vi "SVFA Frequency Response Subset (Real-Im).vi"(0 "stimulus signal X [EUx]":waveform(dbl)={"t0"=timestamp(0 s since 1904-01-01), "dt"=1e-05, "Y"=[]}, 1 "response signal Y [EUy]":waveform(dbl)={"t0"=timestamp(0 s since 1904-01-01), "dt"=1e-05, "Y"=[]}, 2 "window":T9=1 items=["None"=0, "Hanning"=1, "Hamming"=2, "Blackman-Harris"=3, "Exact Blackman"=4, "Blackman"=5, "Flat Top"=6, "4 Term B-Harris "=7, "7 Term B-Harris"=8, "Low Sidelobe"=9, "Force - Exponential"=10, "Blackman Nuttall"=11, "Triangle"=30, "Bartlett-Hanning"=31, "Bohman"=32, "Parzen"=33, "Welch"=34, "Kaiser"=60, "Dolph-Chebyshev"=61, "Gaussian"=62], 3 "frequency range":T7={"start frequency"=1000.0, "stop frequency"=5000.0} {"stop frequency" min=0.0 format="%.2f"; "start frequency" min=0.0 format="%.2f"}, 5 "error in (no error)":errorcluster, 6 "FRF mode":enum16{"H1", "H2", "H3"}(ring), 7 "averaging parameters":T10={"averaging mode"=enum."No averaging", "weighting mode"=enum."Exponential", "number of averages"=10, "linear mode"=enum."One shot"}, 8 "force/exp settings":T8={"force window [%]"=50.0, "exp window [%]"=10.0} {"exp window [%]" min=0.0 max=100.0 format="%.2f"; "force window [%]" min=0.0 max=100.0 format="%.2f"}, 9 "restart averaging (F)":bool) -> (11 "averaging done":bool, 12 "coherence":cluster{"f0":dbl, "df":dbl, "coherence":dbl[]}={"f0"=nan, "df"=inf, "coherence"=[]} {"coherence" format="%.2f"; "df" format="%.2f"; "f0" format="%.2f"}, 13 "averages completed":dbl, 14 "real part [EUy/EUx rms]":cluster{"f0":dbl, "df":dbl, "real part":dbl[]}={"f0"=nan, "df"=inf, "real part"=[]} {"real part" format="%.2f"; "df" format="%.2f"; "f0" format="%.2f"}, 16 "imaginary part [EUy/EUx rms]":T11={"f0"=nan, "df"=inf, "imaginary part"=[]} {"imaginary part" format="%.2f"; "df" format="%.2f"; "f0" format="%.2f"}, 17 "unit label":string=" rms", 18 "spectrum info":T1={"channel name"="", "description"="", "x-axis units"=1, "spectral info"={"spectrum type"=enum."Power [Magnitude^2]", "linear/dB"=enum."linear", "window"=0, "window size"=0, "FFT size"=0}, "engineering units"=0, "custom label"="", "dB reference [EU]"=0.0, "peak units"=enum."rms", "weighting filter"=0, "spectral density?"=FALSE, "unit label"="", "spectrum skewed?"=FALSE, "complimentary spectrum units"=enum."none"} {"x-axis units" items=["Time (s)"=0, "Frequency-CB (Hz)"=1, "Frequency-CPB (Hz)"=1248, "Frequency-Arbitrary (Hz)"=2357, "Quefrency (s)"=2, "Revolutions (rev)"=3, "Order"=4, "Speed (RPM)"=11, "Speed (rad/s)"=21, "Index"=65535]; "weighting filter" items=["Linear", "A-weighting", "B-weighting", "C-weighting", "ITU-R 468-4", "Dolby", "CCITT", "C-message", "Wb", "Wc", "Wd", "We", "Wf", "Wh", "Wj", "Wk", "Wm", "AES17 20 kHz lowpass", "AES17 40 kHz lowpass", "AES17 20 kHz highpass", "AES17 40 kHz highpass"]; "dB reference [EU]" format="%.2f"; "engineering units" items=["custom..."=0, "V"=1, "A"=21, "C"=30, "pC"=31, "s"=32, "-"=29, "Pa"=2, "N"=20, "g"=3, "m/s^2"=4, "m/s"=5, "m"=6, "mm/s"=12, "mm"=13, "micron/s"=14, "micron"=15, "in/s^2"=7, "in/s"=8, "in"=9, "mil/s"=10, "mil"=11, "rad/s^2"=16, "rad/s"=17, "rad"=18, "deg/s^2"=26, "deg/s"=27, "deg"=28, "RPM"=22, "cycle/s^2"=23, "Hz"=24, "cycle"=25, "strain"=19]; "spectral info"."window" items=["None "=0, "Hanning"=1, "Hamming"=2, "Blackman-Harris"=3, "Exact Blackman"=4, "Blackman"=5, "Flat Top"=6, "4 Term B-Harris "=7, "7 Term B-Harris"=8, "Low Sidelobe"=9, "Force - Exponential"=10, "Gaussian"=62]}, 19 "error out":errorcluster)   [LabVIEW 2017]
doc: "Computes a subset of the frequency response and of the coherence of <B>stimulus signal X [EUx]</B> and <B>response signal Y [EUy]</B>. The subset is defined by <B>frequency range</B>. Results are returned in coherence, real part, and imaginary part."
uses:
  <vilib>/addons/_NISVFA/_Shared subVIs/Controls/svc_Window [Dual FFT].ctl
  <vilib>/addons/_NISVFA/_Shared subVIs/Controls/svc_Spectrum Info.ctl
  <vilib>/addons/_NISVFA/_Shared subVIs/Controls/svc_X-Axis Units.ctl
  <vilib>/addons/_NISVFA/_Shared subVIs/Controls/svc_Spectrum Type.ctl
  <vilib>/addons/_NISVFA/_Shared subVIs/Controls/svc_Engineering Units Text Ring.ctl
  <vilib>/addons/_NISVFA/_Shared subVIs/Controls/svc_Weighting Filter Text Ring.ctl
  <vilib>/addons/_NISVFA/_Shared subVIs/Controls/svc_Complimentary Spectrum Units.ctl
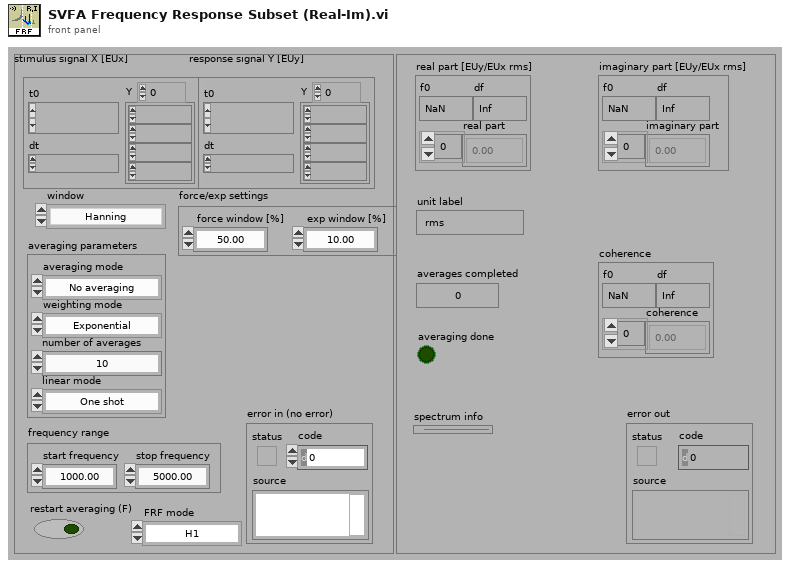
[diagram p1: front panel]
types:
  T1 = typedef "svc_Spectrum Info.ctl" = cluster{"channel name":string, "description":string, "x-axis units":T2, "spectral info":cluster{"spectrum type":T3, "linear/dB":enum16{"linear", "dB"}, "window":u16, "window size":i32, "FFT size":i32}, "engineering units":T4, "custom label":string, "dB reference [EU]":dbl, "peak units":enum16{"rms", "peak", "peak-peak"}, "weighting filter":T5, "spectral density?":bool, "unit label":string, "spectrum skewed?":bool, "complimentary spectrum units":T6}
  T2 = typedef "svc_X-Axis Units.ctl" = u16
  T3 = typedef "svc_Spectrum Type.ctl" = enum16{"FFT Spectrum [complex]", "Amplitude [Magnitude]", "Power [Magnitude^2]", "Cross Spectrum [complex]", "Frequency Response [Complex]"}
  T4 = typedef "svc_Engineering Units Text Ring.ctl" = u16
  T5 = typedef "svc_Weighting Filter Text Ring.ctl" = u16
  T6 = typedef "svc_Complimentary Spectrum Units.ctl" = enum16{"none", "radians", "degrees", "cycles", "imaginary"}
  T7 = cluster{"start frequency":dbl, "stop frequency":dbl}
  T8 = cluster{"force window [%]":dbl, "exp window [%]":dbl}
  T9 = typedef "svc_Window [Dual FFT].ctl" = u32
  T10 = cluster{"averaging mode":enum16{"No averaging", "Vector averaging", "RMS averaging", "Peak hold"}, "weighting mode":enum16{"Linear", "Exponential"}, "number of averages":u32, "linear mode":enum16{"One shot", "Auto restart"}}
  T11 = cluster{"f0":dbl, "df":dbl, "imaginary part":dbl[]}
  T12 = enum16{"Cross spectrum", "Frequency response", "Coherent output power"}
  T13 = enum16{"Restart processing", "Continue processing", "Skip processing"}
  T14 = cluster{"f0":dbl, "df":dbl, "complex spectrum":cdb[]}
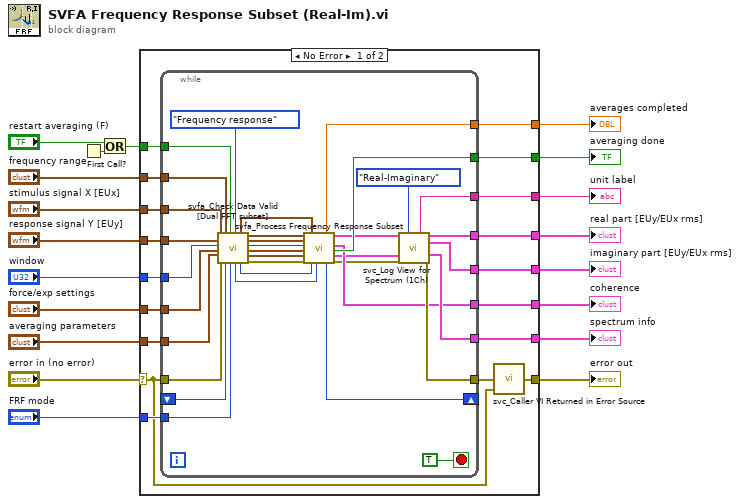
[diagram p0: block diagram]
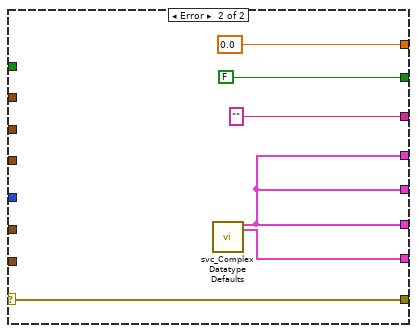
[diagram p2: hidden frame]
diagram:
  n1 = First Call?() -> (First Call?: T/F=w3:bool)
  n2 = Or(x="restart averaging (F)", y=w3) -> (x .or. y?=w1:bool)
  n3 = case shown="No Error" "error in (no error)" {
    selector: "error in (no error)" -> [w20 w77]
    tunnel: "averaging parameters" -> [w31 _]
    tunnel: "window" -> [w33 _]
    tunnel: "force/exp settings" -> [w32 _]
    tunnel: "stimulus signal X [EUx]" -> [w37 _]
    tunnel: "response signal Y [EUy]" -> [w34 _]
    tunnel: [w26 w73] -> w8
    tunnel: [w23 w73] -> w4
    tunnel: [w22 w73] -> w5
    tunnel: [w21 w77] -> w6
    tunnel: [w28 0.0 ("averages completed")] -> w11
    tunnel: w1 -> [w35 _]
    tunnel: "frequency range" -> [w36 _]
    tunnel: [w30 FALSE ("averaging done")] -> w10
    tunnel: "FRF mode" -> [w29 _]
    tunnel: [w27 "" ("unit label (mag or real)")] -> w9
    tunnel: [w25 w72] -> w7
    frame No Error {
      n4 = while {
        tunnel: [w40] -> w22
        tunnel: [w43] -> w23
        tunnel: [w44] -> w24
        tunnel: [w45] -> w25
        tunnel: [w46] -> w26
        tunnel: [w47] -> w27
        tunnel: [w48] -> w28
        tunnel: w29 -> [w51]
        tunnel: [w56] -> w30
        tunnel: w20 -> [w63]
        tunnel: w31 -> [w64]
        tunnel: w32 -> [w65]
        tunnel: w33 -> [w66]
        tunnel: w34 -> [w67]
        tunnel: w35 -> [w68]
        tunnel: w36 -> [w69]
        tunnel: w37 -> [w70]
        shift-left: _ -> [w54]
        shift-right: [w52] -> _
        stop <- TRUE stop-if-true
        n5 = call <vilib>:"svfa_Check Data Valid [Dual FFT subset].vi"("stimulus [X]"=w70, "response [Y]"=w67, "window"=w66, "force/exp settings"=w65, "averaging parameters"=w64, "error in (no error)"=w63, "frequency range"=w69, "processing control in"=w54, "restart averaging (F)"=w68, "FRF mode"=w51, "measurement"=T12."Frequency response") -> ("dup FRF mode"=w50:enum16{"H1", "H2", "H3"}, "dup frequency range"=w49:T7, "processing control out"=w53:T13, "dup stimulus [X]"=w62:waveform(dbl), "dup response [Y]"=w61:waveform(dbl), "window"=w60:u16, "dup force/exp settings"=w59:T8, "dup averaging parameters"=w58:T10, "error out"=w57:errorcluster)
        n6 = call <vilib>:"svfa_Process Frequency Response Subset.vi"("Windowed signal [X]"=w62, "Windowed signal [Y]"=w61, "window (includes Force_Exp)"=w60, "force/exp settings"=w59, "averaging parameters"=w58, "error in (no error)"=w57, "Spectrum Settings"=w49, "processing control"=w53, "FRF mode"=w50) -> ("averages completed"=w48:dbl, "processing control"=w52:T13, "complex frequency response"=w55:T14, "Coherence"=w40:cluster{"f0":dbl, "df":dbl, "Spectrum":dbl[]}, "averaging done"=w56:bool, "spectrum info"=w38:T1, "error out"=w39:errorcluster)  [unwired: 4 in]
        n7 = call <vilib>:"svc_Log View for Spectrum (1Ch).vi"("complex spectrum"=w55, "View"=enum16{"Mag-Phase", "Real-Imaginary"}."Real-Imaginary", "spectrum info in"=w38, "error in (no error)"=w39) -> ("unit label [mag or real]"=w47:string, "magnitude or real"=w46:cluster{"f0":dbl, "df":dbl, dbl[]}, "phase or imag"=w43:cluster{"f0":dbl, "df":dbl, dbl[]}, "spectrum info out"=w45:T1, "error out"=w44:errorcluster)  [unwired: 6 in, 1 out]
      }
      n8 = call <vilib>:"svc_Caller VI Returned in Error Source.vi"("warning input to caller"=w20, "error in (no error)"=w24) -> ("error out"=w21:errorcluster)  [unwired: 3 in]
    }
    frame Error {
      n9 = call <vilib>:"svc_Complex Datatype Defaults.vi"() -> ("empty spectrum"=w73:cluster{"f0":dbl, "df":dbl, "magnitude":dbl[]}, "dead spectrum info"=w72:T1)  [unwired: 11 in, 7 out]
    }
  }
  "error out" <- w6
  "real part [EUy/EUx rms]" <- w8
  "imaginary part [EUy/EUx rms]" <- w4
  "averaging done" <- w10
  "averages completed" <- w11
  "coherence" <- w5
  "unit label" <- w9
  "spectrum info" <- w7
